vi "TeleOP(Ramps).vi"(10 "Match Info":T1={"Autonomous Elapsed Seconds"=0.0, "TeleOp Elapsed Seconds"=0.0, "Disabled Elapsed Seconds"=0.0, "Visited Autonomous"=FALSE, "Visited TeleOp"=FALSE, "Visited Disabled"=FALSE, "Autonomous Settings"={"Autonomous Style"=enum."Independent", "VI Refnum"=refnum}}, 11 "Call Context":T2) -> ()   [LabVIEW 2017]
doc: "This VI is called for each enabled TeleOp packet received from the DS. It is typically used to read from joysticks and other inputs and update I/O or setpoints for timed control loops. It should complete and return within 20 milliseconds or risk missing DS packets."
uses:
  <vilib>/Rock Robotics/WPI/DriverStation/WPI_DriverStationDerivedRobotMode.ctl
  <vilib>/Rock Robotics/WPI/DriverStation/WPI_DriverStationMatch Info.ctl
  <vilib>/Rock Robotics/WPI/Utilities/WPI_GetSetVariantRefNum.vi
  <vilib>/Rock Robotics/Network Tables/NT Write Boolean Array.vi
  <vilib>/Rock Robotics/Network Tables/NT Write Numeric Array.vi
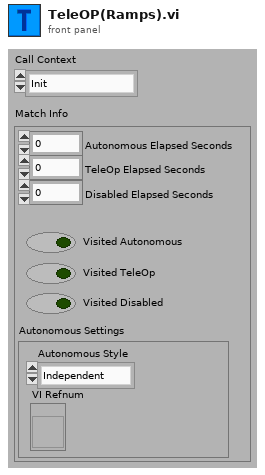
[diagram p1: front panel]
types:
  T1 = typedef "WPI_DriverStationMatch Info.ctl" = cluster{"Autonomous Elapsed Seconds":dbl, "TeleOp Elapsed Seconds":dbl, "Disabled Elapsed Seconds":dbl, "Visited Autonomous":bool, "Visited TeleOp":bool, "Visited Disabled":bool, "Autonomous Settings":cluster{"Autonomous Style":enum16{"Iterative", "Independent"}, "VI Refnum":refnum<vi>}}
  T2 = typedef "WPI_DriverStationDerivedRobotMode.ctl" = enum16{"Init", "Execute", "Stop"}
  T3 = typedef "WPI_JoystickDevRef.ctl" = cluster{"Device":T4}
  T4 = typedef "WPI_JoystickDeviceEnum.ctl" = enum16{"USB 0", "USB 1", "USB 2", "USB 3", "USB 4", "USB 5"}
  T5 = typedef "Command Status Info.ctl" = cluster{"Name":string, "Status":T6, "notifier out":T7}
  T6 = typedef "Completion Status.ctl" = enum16{"Successful", "Aborted", "Incomplete"}
  T7 = typedef "Completion Notifier.ctl" = refnum<notifier>
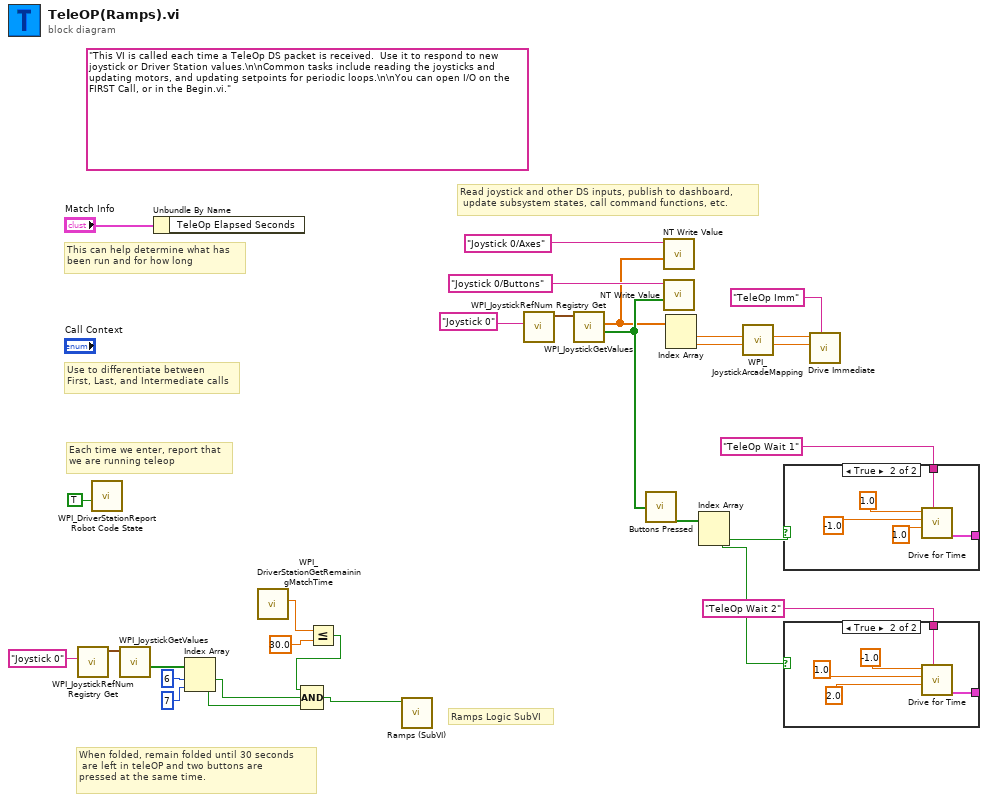
[diagram p0: block diagram]
diagram:
  (unwired) "This VI is called each time a TeleOp DS packet is received.  Use it to respond to new joystick or Driver Station values.\n\nCommon tasks include reading the joysticks and updating motors, and updating setpoints for periodic loops.\n\nYou can open I/O on the FIRST Call, or in the Begin.vi."
  # "Ramps Logic SubVI"
  # "When folded, remain folded until 30 seconds\n are left in teleOP and two buttons are \npressed at the same time."
  # "Read joystick and other DS inputs, publish to dashboard,\n update subsystem states, call command functions, etc."
  # "Each time we enter, report that\nwe are running teleop"
  # "Use to differentiate between\nFirst, Last, and Intermediate calls"
  # "This can help determine what has\nbeen run and for how long"
  n1 = call <vilib>:"WPI_JoystickRefNum Registry Get.vi"("refnum name"="Joystick 0") -> ("JoystickDevRef"=w11:T3)  [unwired: 9 in, 1 out]
  n2 = call <vilib>:"WPI_DriverStationReport Robot Code State.vi"("TeleOp"=TRUE ("Autonomous")) -> ()  [unwired: 10 in, 1 out]
  n3 = call <vilib>:"WPI_JoystickGetValues.vi"("JoystickDevRef"=w11) -> ("Buttons"=w7:bool[])  [unwired: 6 in, 4 out]
  n4 = Unbundle By Name("Match Info") -> ()  [unwired: 1 out]
  n5 = Index Array(array=w7, index #1=6 ("index"), index #2=7 ("index")) -> (element #1=w3:bool, element #2=w2:bool)
  n6 = call <vilib>:"WPI_DriverStationGetRemainingMatchTime.vi"() -> ("Match Time(s)"=w6:sgl)  [unwired: 10 in, 1 out]
  n7 = Less Or Equal?(x=w6, y=sgl 30.0) -> (x <= y?=w4:bool)
  n8 = Compound Arithmetic op=AND(w4, w3, w2) -> (w1:bool)
  n9 = call "Ramps (SubVI).vi"("canRun?"=w1) -> ()  [unwired: 10 in, 1 out]
  n10 = call <vilib>:"WPI_JoystickRefNum Registry Get.vi"("refnum name"="Joystick 0") -> ("JoystickDevRef"=w26:T3)  [unwired: 1 in, 9 out]
  n11 = call <vilib>:"WPI_JoystickGetValues.vi"("JoystickDevRef"=w26) -> ("Buttons"=w14:bool[], "Axes"=w13:dbl[])  [unwired: 6 in, 3 out]
  n12 = call "Buttons Pressed.vi"("Button Values"=w14) -> ("Button Presses"=w22:bool[])
  n13 = call-poly <vilib>:"NT Write Value.vi"("Numeric Array"=w13, "Name"="Joystick 0/Axes") -> ()  [unwired: 9 in, 1 out]
  n14 = call-poly <vilib>:"NT Write Value.vi"("Boolean Array"=w14, "Name"="Joystick 0/Buttons") -> ()  [unwired: 9 in, 1 out]
  n15 = Index Array(array=w13) -> (element #1=w17:dbl, element #2=w16:dbl)  [unwired: 2 in]
  n16 = Index Array(array=w22) -> (element #1=w21:bool, element #2=w20:bool)  [unwired: 2 in]
  n17 = call <vilib>:"WPI_JoystickArcadeMapping.vi"("Y axis value"=w16, "X axis value"=w17) -> ("Right Motor Value"=w18:dbl, "Left Motor Value"=w19:dbl)  [unwired: 8 in]
  n18 = case shown="True" w21 {
    tunnel: [_ w33] -> _
    tunnel: "TeleOp Wait 1" ("Description") -> [_ w32]
    frame False {
    }
    frame True {
      n19 = call "Drive for Time.vi"("Description"=w32, "Seconds"=1.0, "Right Speed"=-1.0, "Left Speed"=1.0) -> ("Command Info Out"=w33:T5)  [unwired: 6 in, 1 out]
    }
  }
  n20 = case shown="True" w20 {
    tunnel: [_ w37] -> _
    tunnel: "TeleOp Wait 2" ("Description") -> [_ w36]
    frame False {
    }
    frame True {
      n21 = call "Drive for Time.vi"("Description"=w36, "Seconds"=2.0, "Right Speed"=1.0, "Left Speed"=-1.0) -> ("Command Info Out"=w37:T5)  [unwired: 6 in, 1 out]
    }
  }
  n22 = call "Drive Immediate.vi"("Description"="TeleOp Imm", "Right Setpoint"=w18, "Left Setpoint"=w19) -> ()  [unwired: 8 in, 1 out]
